vi "Read ZM_State.vi"(11 "HE_ZM_state in":refnum<class "HE_ZM_state.lvclass">) -> (2 "ZM_State":T1, 3 "HE_ZM_state out":refnum<class "HE_ZM_state.lvclass">)   [LabVIEW 2019, in "Heating.lvlib" / "HE_ZM_state.lvclass"]
uses:
  HE_ZM_state.lvclass
  ctl/ZM_State.ctl
  HE_ZM_state.lvclass/HE_ZM_state.ctl
  Heating.lvlib
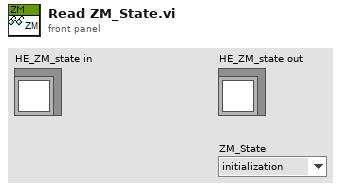
[diagram p1: front panel]
types:
  T1 = typedef "Heating.lvlib/ZM_State.ctl" = enum8{"initialization", "stop", "start_cmd", "contactor_on_cmd", "heating", "on", "stop_cmd", "power_down", "contactor_off_cmd", "cooling", "restart_delay"}
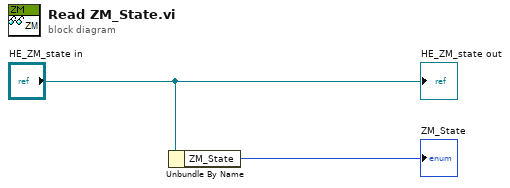
[diagram p0: block diagram]
diagram:
  n1 = Unbundle By Name("HE_ZM_state in") -> ("ZM_State"=→"ZM_State":T1)
  "HE_ZM_state out" <- "HE_ZM_state in"
